vi "main.vi"() -> ()   [LabVIEW 2024, in "CLZ_to_ComicVine.lvlib"]
uses:
  CLZ_to_ComicVine.lvlib
  typedefs/CLZ_series.ctl
  comic_manager/manager_daemon/type_defs/VolumeData--cluster.ctl
  CV_Shared_Library/volume.type--enum.ctl
  <vilib>/addons/_JKI Toolkits/State Machine/_JKI_lib_State_Machine.llb/Select State(s)_err__jki_lib_state_machine.vi
  <vilib>/addons/_JKI Toolkits/State Machine/_JKI_lib_State_Machine.llb/Periodic Trigger__ogtk__JKI-SM__jki_lib_state_machine.vi
  CV_Shared_Library/CV_Shared_Library.lvlib
  comic_manager/manager_daemon/manager_daemon.lvclass
panel:
  in  "CV Volumes":i32(listbox)
  in  "CLZ Volumes":i32(listbox)
  in  "Load Files":bool
  in  "Exit":bool
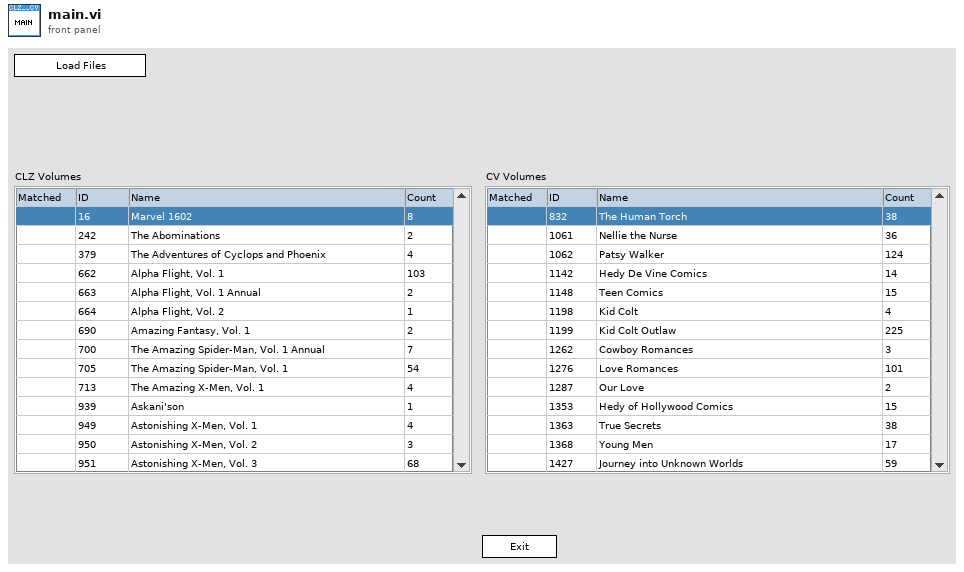
[diagram p1: front panel]
types:
  T1 = enum32{"Invalid", "Standard", "Closed", "Hidden", "Minimized", "Maximized"}
  T2 = enum32{"invalid app kind", "Development System", "Run Time System", "Student Edition", "Embedded LabVIEW", "Evaluation", "Custom"}
  T3 = typedef "CLZ_to_ComicVine.lvlib/CLZ_series.ctl" = cluster{"name":string, "id":i32, "earliest date":timestamp, "latest date":timestamp, "issue numbers":set{i32}}
  T4 = typedef "manager_daemon.lvclass/VolumeData--cluster.ctl" = cluster{"name":string, "sortable_name":string, "aliases":string[], "description":string, "site_detail_url":string, "count_of_issues":i32, "start_year":i32, "publisher_id":i32, "issue_ids":i32[], "date_last_updated":timestamp, "volume":i32, "cv_id":string, "volume type":T5, "source_path":path}
  T5 = typedef "CV_Shared_Library.lvlib/volume.type--enum.ctl" = enum16{"Ongoing", "Limited Series", "Annual", "One Shot", "Reprint/Document", "Star Comics", "Epic Comics"}
  T6 = cluster{"Core":cluster{"Current VI Reference":refnum<vi>, "Close Panel on Exit?":bool}, "CLZ report path":path, "clz series map":map{i32, T3}, "CV binary path":path, "cv volume map":map{i32, T4}, "matched volumes set":set{cluster{"CLZ ID":i32, "CV ID":i32}}}
  T7 = cluster{"Current VI Reference":refnum<vi>, "Close Panel on Exit?":bool}
  T8 = typedef "CLZ_to_ComicVine.lvlib/CLZ_comic.ctl" = cluster{"Series":string, "Core SeriesID":i32, "Core ComicID":i32, "Issue":string, "Issue Nr":i32, "Release Date":timestamp, "Barcode":string, "Cover Price":dbl, "CovrPrice Value":dbl, "Purchase Price":dbl, "Characters":string[]}
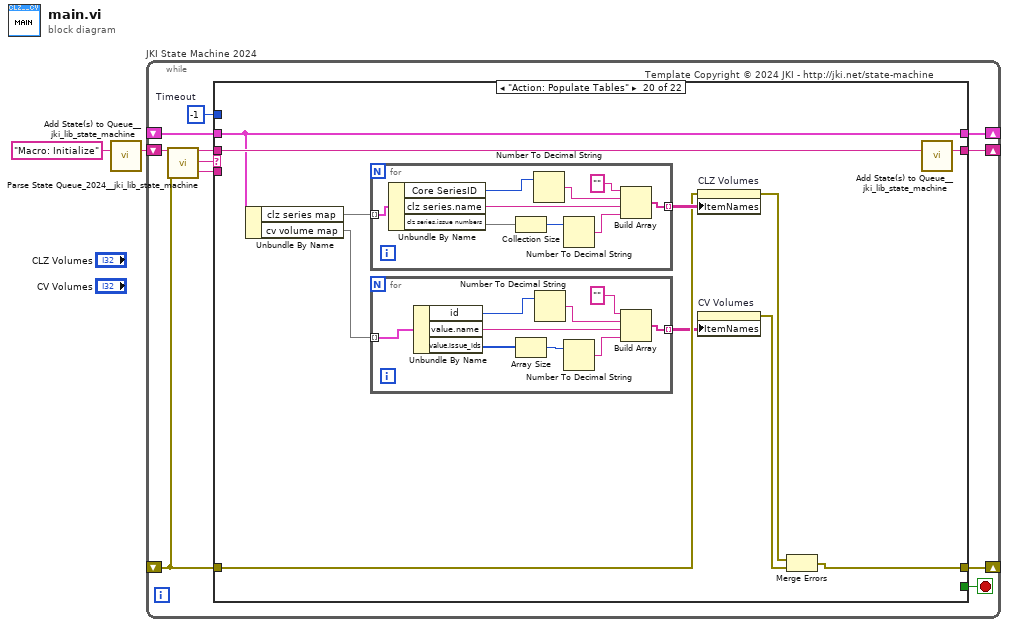
[diagram p0: block diagram]
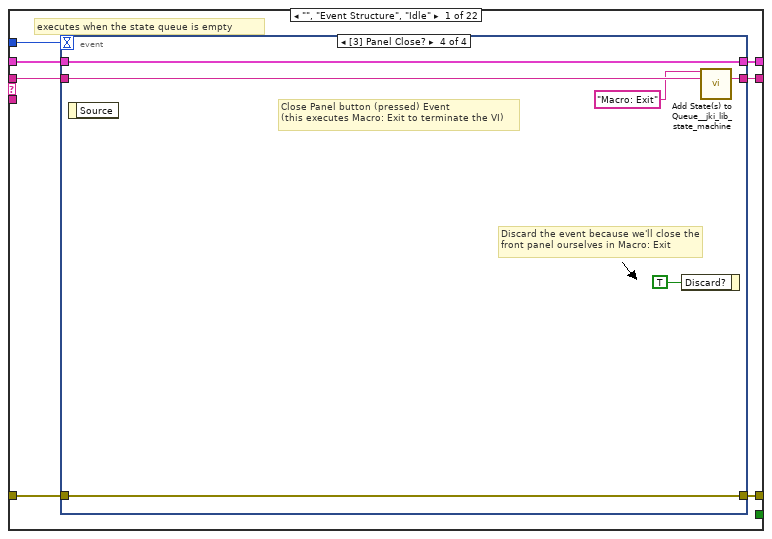
[diagram p2: hidden frame]
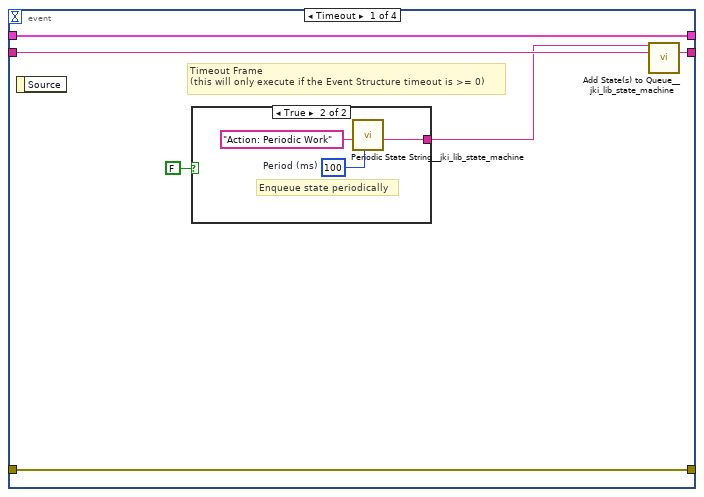
[diagram p3: hidden frame]
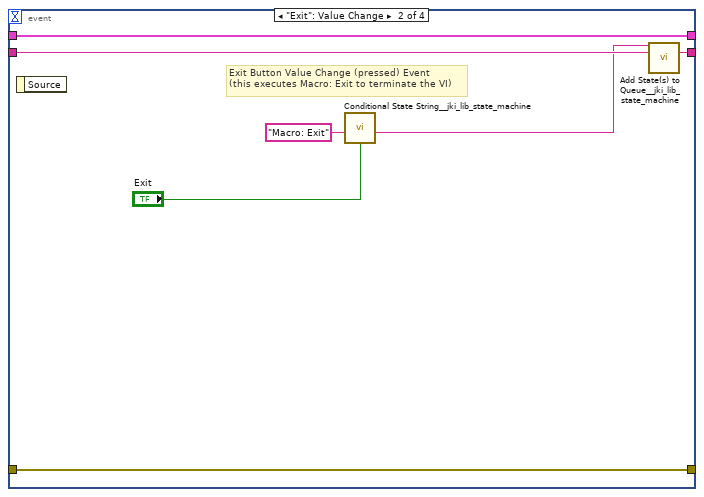
[diagram p5: hidden frame]
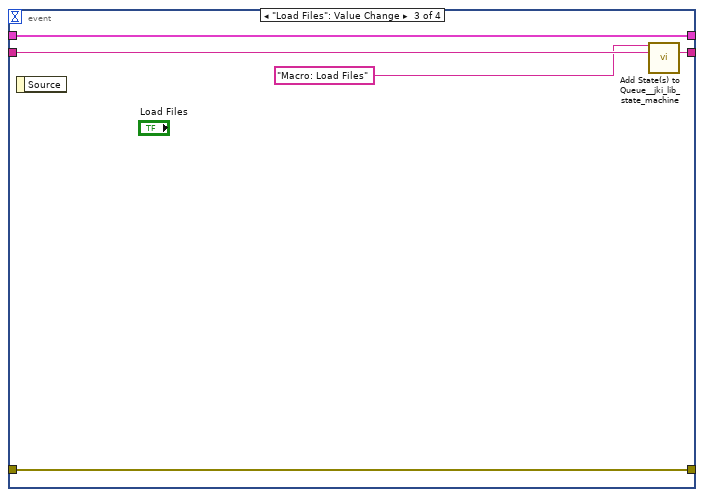
[diagram p6: hidden frame]
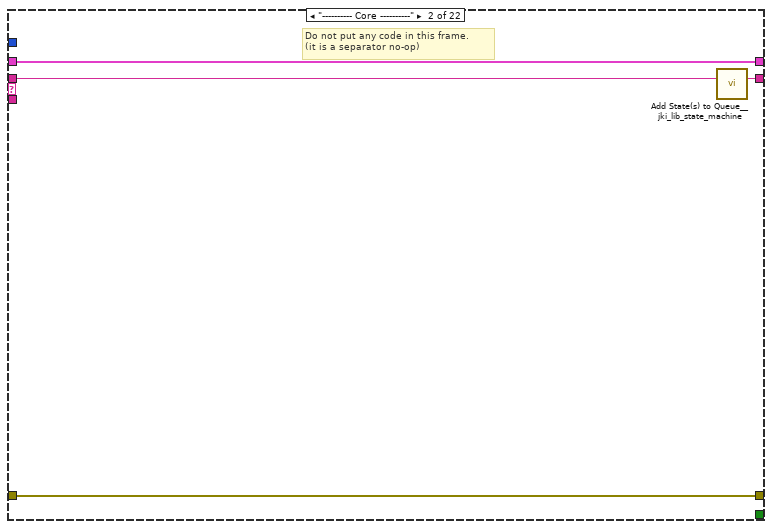
[diagram p7: hidden frame]
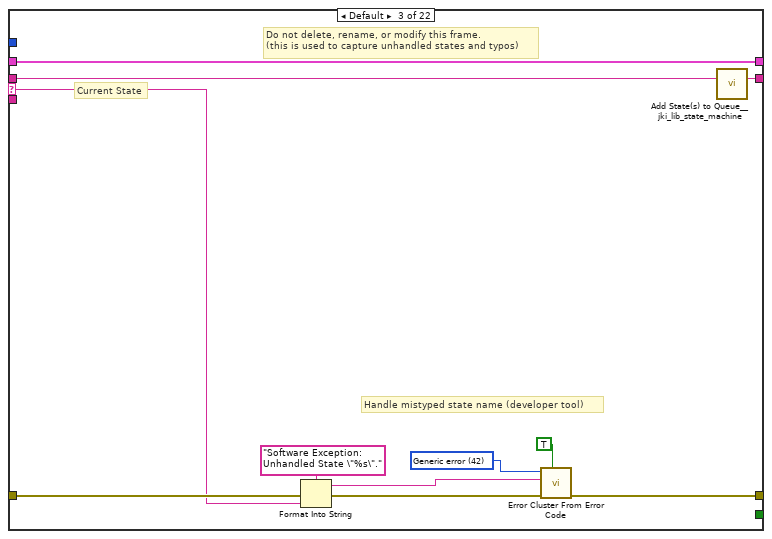
[diagram p8: hidden frame]
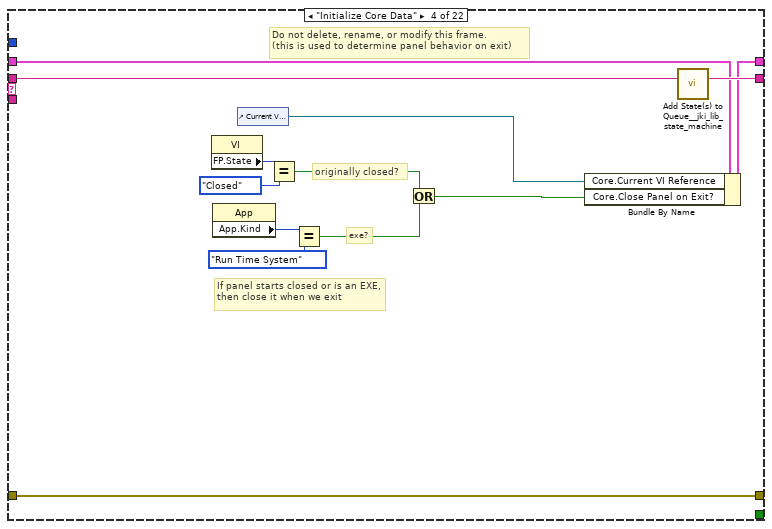
[diagram p9: hidden frame]
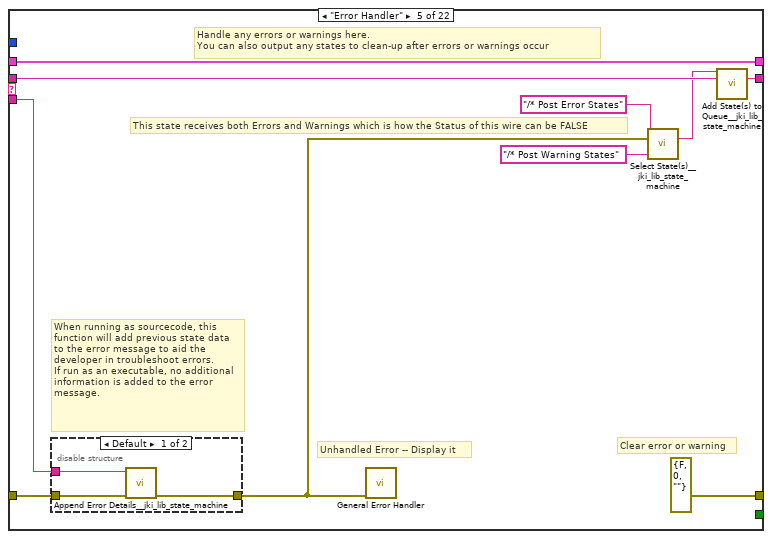
[diagram p10: hidden frame]
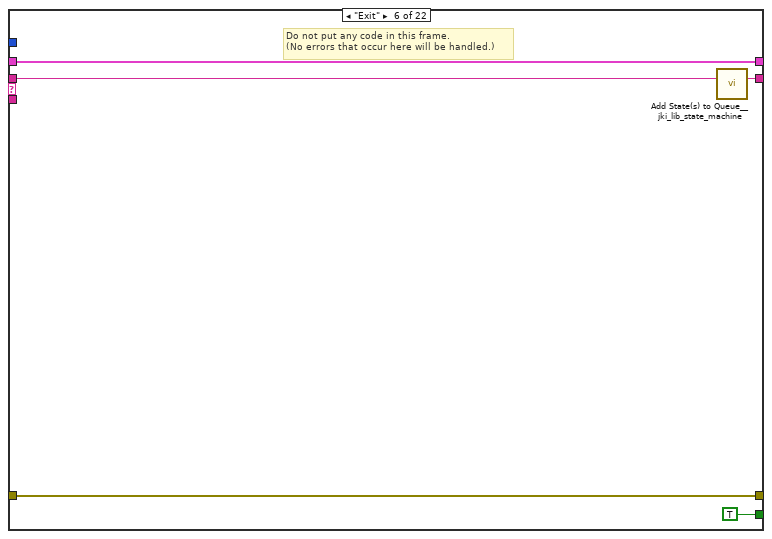
[diagram p12: hidden frame]
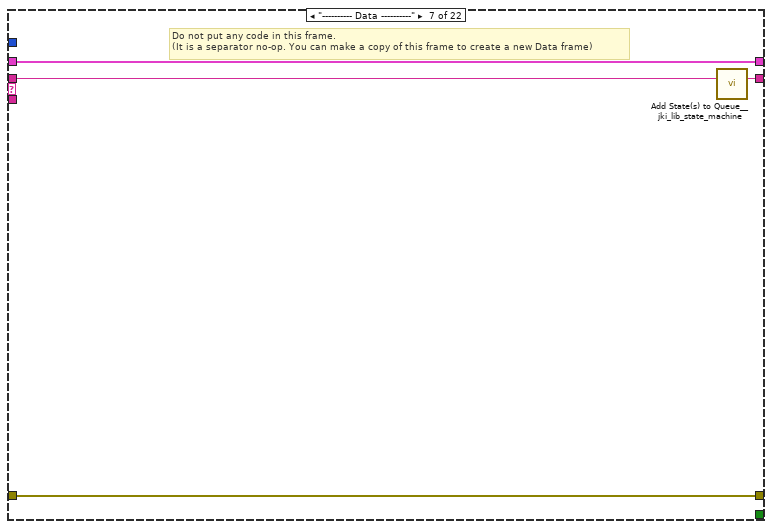
[diagram p13: hidden frame]
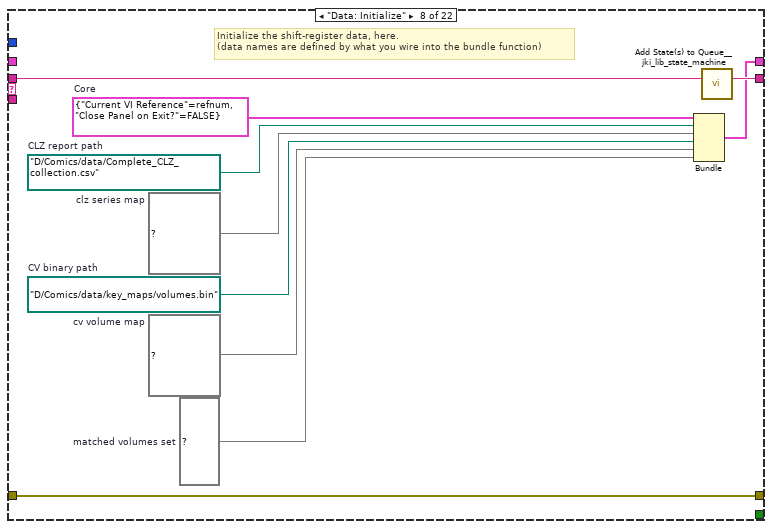
[diagram p14: hidden frame]
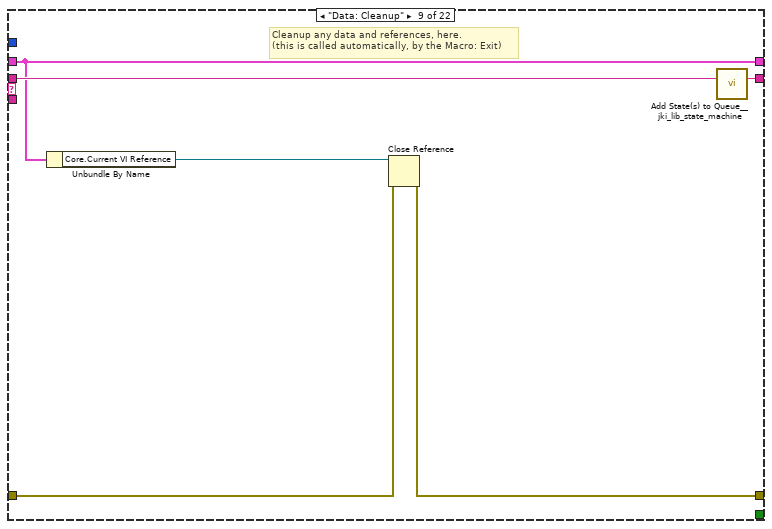
[diagram p15: hidden frame]
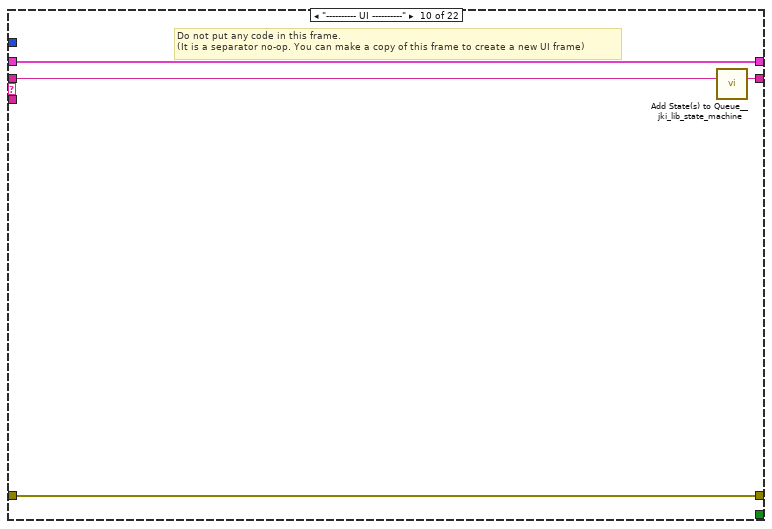
[diagram p16: hidden frame]
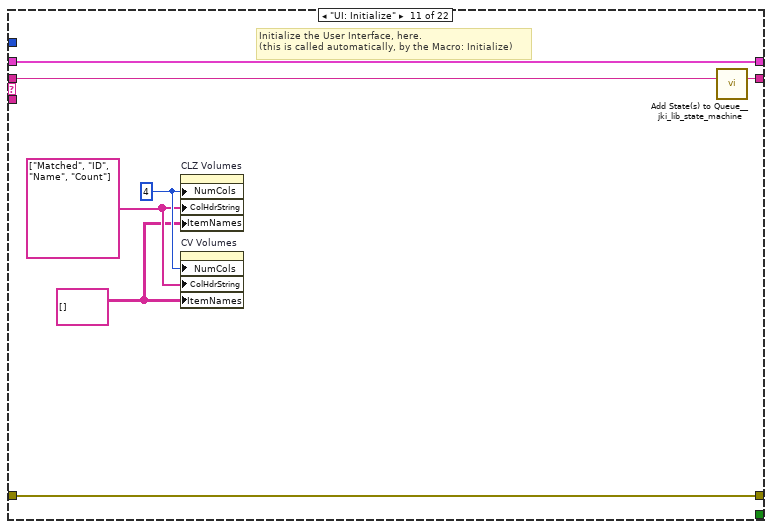
[diagram p17: hidden frame]
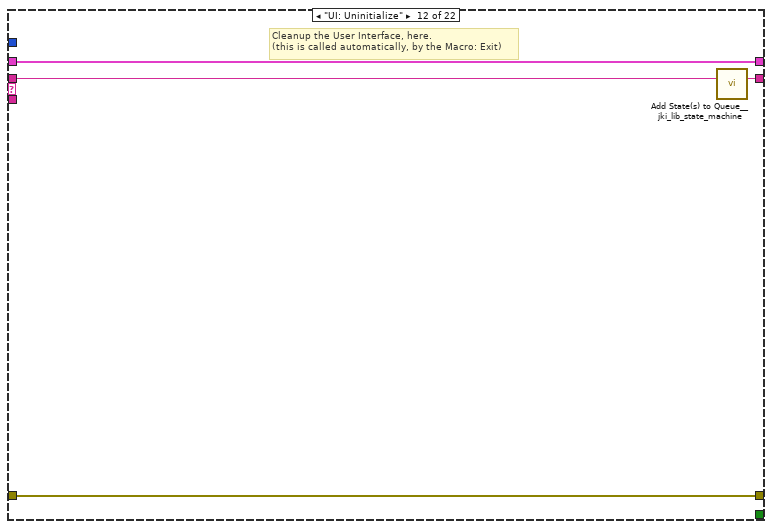
[diagram p18: hidden frame]
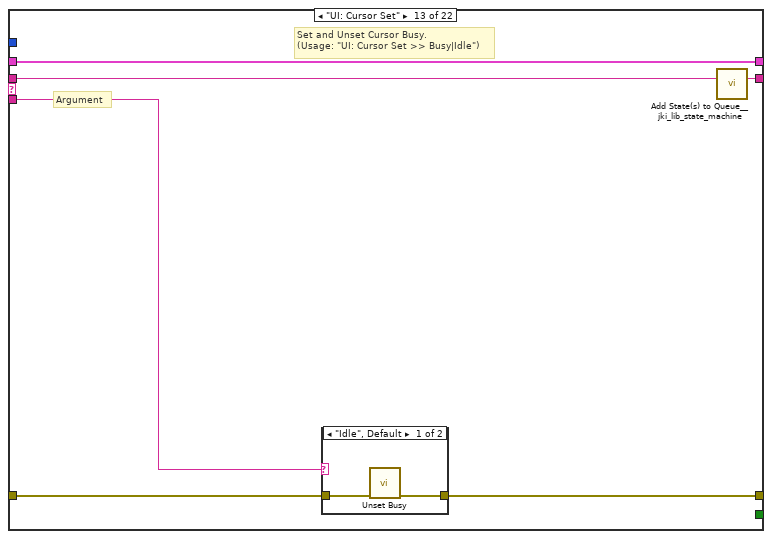
[diagram p19: hidden frame]
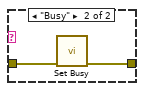
[diagram p20: hidden frame]
diagram:
  n1 = call <vilib>:"Add State(s) to Queue__jki_lib_state_machine.vi"("State(s) in (\"\")"="Macro: Initialize") -> ("States Out"=w2:string)  [unwired: 14 in]
  n2 = while "JKI State Machine 2024" {
    shift-right: [w6] -> _
    shift-left: _ -> [w5]
    shift-right: [w9] -> _
    shift-left: _ -> [w3]
    shift-right: [w8] -> _
    shift-left: w2 -> [w10]
    stop <- w7 stop-if-true
    w4 = -1  # Timeout
    # "Template Copyright © 2024 JKI - http://jki.net/state-machine"
    n3 = call <vilib>:"Parse State Queue_2024__jki_lib_state_machine.vi"("State Queue"=w10, "Error In (no error)"=w3) -> ("Remaining States"=w12:string, "Current State"=w13:string, "Arguments"=w11:string)  [unwired: 11 in]
    n4 = case shown="\"Action: Populate Tables\"" w13 {
      selector: w13 -> [_ _ w52 _ _ _ _ _ _ _ _ _ _ _ _ _ _ _ _ _ _ _]
      tunnel: w12 -> [w20 w51 w56 w75 w85 w94 w98 w108 w114 w118 w125 w129 w135 w146 w215 w220 w225 w234 w238 w249 w276 w282]
      tunnel: w11 -> [_ _ _ _ w80 _ _ _ _ _ _ _ w130 w140 _ _ _ _ _ _ _ _]
      tunnel: w5 -> [w18 w48 w54 w68 w82 w92 w95 _ w109 w115 w123 w127 w133 w142 w212 w217 w222 w232 w235 w247 w271 w280]
      tunnel: [w17 w49 w58 w72 errorcluster {"status"=FALSE, "code"=0, "source"=""} ("error out") w91 w96 w105 w110 w116 w122 w126 w131 w143 w213 w218 w223 w229 w236 w239 w273 w279] -> w9
      tunnel: w3 -> [w14 w49 w57 w72 w81 w91 w96 w105 w111 w116 w122 w126 w132 w144 w213 w218 w223 w229 w236 w244 w272 w278]
      tunnel: [w19 w50 w55 w74 w84 w93 w97 w107 w113 w117 w124 w128 w134 w145 w214 w219 w224 w233 w237 w248 w275 w281] -> w8
      tunnel: [_ _ _ _ _ TRUE _ _ _ _ _ _ _ _ _ _ _ _ _ _ _ _] -> w7
      tunnel: [w16 w48 w54 w73 w82 w92 w95 w106 w109 w115 w123 w127 w133 w142 w212 w217 w222 w232 w235 w247 w270 w277] -> w6
      tunnel: w4 -> [w15 _ _ _ _ _ _ _ _ _ _ _ _ _ _ _ _ _ _ _ _ _]
      frame "", "Event Structure", "Idle" {
        # "executes when the state queue is empty"
        n5 = event shown="[3] Panel Close?" {
          selector: _ -> [_ _ _ _]
          dyn-events: _ -> [_ _ _ _]
          timeout: w15 -> [_ _ _ _]
          tunnel: w20 -> [w26 w36 w41 w47]
          tunnel: [w25 w35 w40 w46] -> w19
          tunnel: w18 -> [w23 w33 w38 w44]
          tunnel: [w24 w34 w39 w45] -> w17
          tunnel: w14 -> [w24 w34 w39 w45]
          tunnel: [w23 w33 w38 w44] -> w16
          event Timeout {
            # "Timeout Frame\n(this will only execute if the Event Structure timeout is >= 0)"
            n6 = event-data() -> ()  [unwired: 1 in, 1 out]
            n7 = case shown="True" FALSE {
              tunnel: [_ w29] -> w22
              frame False {
              }
              frame True {
                w27 = u32 100  # Period (ms)
                # "Enqueue state periodically"
                n8 = call <vilib>:"Periodic State String__jki_lib_state_machine.vi"("Period (ms)"=w27, "State"="Action: Periodic Work") -> ("State Out"=w29:string)  [unwired: 9 in]
              }
            }
            n9 = call <vilib>:"Add State(s) to Queue__jki_lib_state_machine.vi"("State(s) in Front (\"\")"=w22, "State(s) in (\"\")"=w26) -> ("States Out"=w25:string)  [unwired: 13 in]
          }
          event "Exit": Value Change {
            # "Exit Button Value Change (pressed) Event\n(this executes Macro: Exit to terminate the VI)"
            n10 = event-data() -> ()  [unwired: 1 in, 1 out]
            n11 = call <vilib>:"Conditional State String__jki_lib_state_machine.vi"("Do State(s)?"="Exit", "State"="Macro: Exit") -> ("State Out"=w30:string)  [unwired: 7 in]
            n12 = call <vilib>:"Add State(s) to Queue__jki_lib_state_machine.vi"("State(s) in Front (\"\")"=w30, "State(s) in (\"\")"=w36) -> ("States Out"=w35:string)  [unwired: 13 in]
          }
          event "Load Files": Value Change {
            n13 = event-data() -> ()  [unwired: 1 in, 1 out]
            n14 = call <vilib>:"Add State(s) to Queue__jki_lib_state_machine.vi"("State(s) in Front (\"\")"="Macro: Load Files", "State(s) in (\"\")"=w41) -> ("States Out"=w40:string)  [unwired: 13 in]
          }
          event Panel Close? {
            # "Discard the event because we'll close the front panel ourselves in Macro: Exit"
            # "Close Panel button (pressed) Event\n(this executes Macro: Exit to terminate the VI)"
            n15 = event-data() -> ()  [unwired: 1 in, 1 out]
            n16 = event-data("Discard?"=TRUE) -> ()  [unwired: 1 in, 1 out]
            n17 = call <vilib>:"Add State(s) to Queue__jki_lib_state_machine.vi"("State(s) in Front (\"\")"="Macro: Exit", "State(s) in (\"\")"=w47) -> ("States Out"=w46:string)  [unwired: 13 in]
          }
        }
      }
      frame "---------- Core ----------" {
        # "Do not put any code in this frame.\n(it is a separator no-op)"
        n18 = call <vilib>:"Add State(s) to Queue__jki_lib_state_machine.vi"("State(s) in (\"\")"=w51) -> ("States Out"=w50:string)  [unwired: 14 in]
      }
      frame Default {
        w61 = 42 items=["No error", "Argument error", "Memory is full", "Out of zone", "End of file", "File already open", "Generic file I/O error", "File not found", "File permission error", "Disk is full", "Duplicate path", "Too many files open", "System feature not enabled", "Resource file not found", "Cannot add resource", "Resource not found", "Image not found", "Image memory error", "Pen does not exist", "Config type invalid", "Config token not found", "Config parse error", "Config memory error", "Bad external code format", "Bad external code offset", "External code not present", "Null window", "Destroy window error", "Null menu", "Print aborted", "Bad print record", "Print driver error", "Windows error during printing", "Memory error during printing", "Print dialog error", "Generic print error", "Invalid device refnum", "Device not found", "Device parameter error", "Device unit error", "Cannot open device", "Device call aborted", "Generic error", "Cancelled by user", "Object ID too low", "Object ID too high", "Object not in heap", "Unknown heap", "Unknown object (invalid DefProc)", "Unknown object (DefProc not in table)", "Message out of range", "Invalid (null) method", "Unknown message", "Manager call not supported", "Bad address", "Network operation in progress", "Network operation timed out", "Connection is busy", "Network attribute not supported", "Network error", "Address in use", "System out of memory", "Connection aborted", "Connection refused", "Not connected", "Already connected", "Connection closed", "Initialization error (interapplication manager)", "Bad occurrence", "Wait on unbound occurrence handler", "Occurrence queue overflow", "Datalog type conflict", "Unused", "Unrecognized type (interapplication manager)", "Memory corrupt", "Failed to make temporary DLL", "Old CIN version", "Drag socket not found", "Failed to load drop-object", "Failed to register OLE object", "Failed to release OLE object", "Format specifier type mismatch", "Unknown format specifier", "Too few format specifiers", "Too many format specifiers", "Scan failed", "Newer CIN version", "Error converting to variant", "Runtime menu error", "Password tampered", "Variant attribute not found", "Incompatible variant data type", "Event data is not available", "Event Store is not present", "Occurrence is not found", "Event Queue is not created", "Event info is not available", "Refnum passed is NULL", "Error retrieving Class GUID", "Error retrieving CoClass GUID", "Error retrieving TypeLib GUID.", "Bad built application magic bytes.", "Specific driver is different from the specific driver associated with the Logical Name.", "There is no session opened to the class driver.", "Max Error", "MAX - Error with config objects", "MAX - Error loading configuration", "MAX - Group not supported"]
        # "Current State"
        # "Do not delete, rename, or modify this frame.\n(this is used to capture unhandled states and typos)"
        # "Handle mistyped state name (developer tool)"
        n19 = Format Into String(format string="Software Exception: Unhandled State \"%s\"." ("message"), error in=w57, w52) -> (resulting string=w60:string, error out=w59:errorcluster)  [unwired: 1 in]
        n20 = call <vilib>:"Error Cluster From Error Code.vi"("show call chain? (False)"=TRUE, "error in (no error)"=w59, "error message (\"\")"=w60, "error code (0)"=w61) -> ("error out"=w58:errorcluster)  [unwired: 5 in]
        n21 = call <vilib>:"Add State(s) to Queue__jki_lib_state_machine.vi"("State(s) in (\"\")"=w56) -> ("States Out"=w55:string)  [unwired: 14 in]
      }
      frame "Initialize Core Data" {
        # "Do not delete, rename, or modify this frame.\n(this is used to determine panel behavior on exit)"
        # "originally closed?"
        # "exe?"
        # "If panel starts closed or is an EXE, then close it when we exit"
        n22 = property class="VI"() -> ("FP.State"=w65:T1)  [unwired: 2 in, 2 out]
        n23 = property class="App"() -> ("App.Kind"=w71:T2)  [unwired: 2 in, 2 out]
        n24 = control-ref of="Current VI Reference"() -> (w66:refnum<vi>)
        n25 = Equal?(x=w65, y=T1."Closed" ("Front Panel Window:State")) -> (x = y?=w63:bool)
        n26 = Equal?(x=w71, y=T2."Run Time System" ("Application:Kind")) -> (x = y?=w69:bool)
        n27 = Or(x=w63, y=w69) -> (x .or. y?=w67:bool)
        n28 = Bundle By Name(cluster=w68, "Core.Current VI Reference"=w66, "Core.Close Panel on Exit?"=w67) -> (w73:T6)
        n29 = call <vilib>:"Add State(s) to Queue__jki_lib_state_machine.vi"("State(s) in (\"\")"=w75) -> ("States Out"=w74:string)  [unwired: 14 in]
      }
      frame "Error Handler" {
        # "When running as sourcecode, this function will add previous state data to the error message to aid the developer in troubleshoot errors.\nIf run as an executable, no additional information is added to the error message."
        # "This state receives both Errors and Warnings which is how the Status of this wire can be FALSE"
        # "Unhandled Error -- Display it"
        # "Handle any errors or warnings here.\nYou can also output any states to clean-up after errors or warnings occur"
        # "Clear error or warning"
        n30 = disable-structure shown="Default" {
          disable-tunnel: w81 -> [w88 w89]
          disable-tunnel: w80 -> [w87 _]
          disable-tunnel: [w86 w89] -> w79
          frame condition #0 (active) {
            n31 = call <vilib>:"Append Error Details__jki_lib_state_machine.vi"("error in (no error)"=w88, "Previous State and Argument(s)"=w87) -> ("error out"=w86:errorcluster)  [unwired: 9 in]
          }
          frame condition #1 {
          }
        }
        n32 = call <vilib>:"General Error Handler.vi"("error in (no error)"=w79) -> ()  [unwired: 10 in, 5 out]
        n33 = call-poly <vilib>:"Select State(s)__jki_lib_state_machine.vi"("State(s) if True (\"\")"="/* Post Error States", "Select"=w79, "State(s) if False (\"\")"="/* Post Warning States") -> ("States Out"=w77:string)  [unwired: 12 in]
        n34 = call <vilib>:"Add State(s) to Queue__jki_lib_state_machine.vi"("State(s) in Front (\"\")"=w77, "State(s) in (\"\")"=w85) -> ("States Out"=w84:string)  [unwired: 13 in]
      }
      frame "Exit" {
        # "Do not put any code in this frame.\n(No errors that occur here will be handled.)"
        n35 = call <vilib>:"Add State(s) to Queue__jki_lib_state_machine.vi"("State(s) in (\"\")"=w94) -> ("States Out"=w93:string)  [unwired: 14 in]
      }
      frame "---------- Data ----------" {
        # "Do not put any code in this frame.\n(It is a separator no-op. You can make a copy of this frame to create a new Data frame)"
        n36 = call <vilib>:"Add State(s) to Queue__jki_lib_state_machine.vi"("State(s) in (\"\")"=w98) -> ("States Out"=w97:string)  [unwired: 14 in]
      }
      frame "Data: Initialize" {
        w99 = set{cluster{"CLZ ID":i32, "CV ID":i32}} {}  # matched volumes set
        w100 = map{i32, T4} {}  # cv volume map
        w101 = path "D:/Comics/data/key_maps/volumes.bin"  # CV binary path
        w102 = map{i32, T3} {}  # clz series map
        w103 = path "D:/Comics/data/Complete_CLZ_collection.csv"  # CLZ report path
        w104 = T7 {"Current VI Reference"=refnum, "Close Panel on Exit?"=FALSE}  # Core
        # "Initialize the shift-register data, here.\n(data names are defined by what you wire into the bundle function)"
        n37 = Bundle("Core"=w104, "CLZ report path"=w103, "clz series map"=w102, "CV binary path"=w101, "cv volume map"=w100, "matched volumes set"=w99) -> (w106:T6)  [unwired: 1 in]
        n38 = call <vilib>:"Add State(s) to Queue__jki_lib_state_machine.vi"("State(s) in (\"\")"=w108) -> ("States Out"=w107:string)  [unwired: 14 in]
      }
      frame "Data: Cleanup" {
        # "Cleanup any data and references, here.\n(this is called automatically, by the Macro: Exit)"
        n39 = Unbundle By Name(w109) -> ("Core.Current VI Reference"=w112:refnum<vi>)
        n40 = Close Reference(reference=w112, error in (no error)=w111) -> (error out=w110:errorcluster)
        n41 = call <vilib>:"Add State(s) to Queue__jki_lib_state_machine.vi"("State(s) in (\"\")"=w114) -> ("States Out"=w113:string)  [unwired: 14 in]
      }
      frame "---------- UI ----------" {
        # "Do not put any code in this frame.\n(It is a separator no-op. You can make a copy of this frame to create a new UI frame)"
        n42 = call <vilib>:"Add State(s) to Queue__jki_lib_state_machine.vi"("State(s) in (\"\")"=w118) -> ("States Out"=w117:string)  [unwired: 14 in]
      }
      frame "UI: Initialize" {
        w119 = string[][] []
        w120 = string[] ["Matched", "ID", "Name", "Count"] ("Row Header Strings[]")
        w121 = u32 4 ("Number of Columns")
        # "Initialize the User Interface, here.\n(this is called automatically, by the Macro: Initialize)"
        n43 = property on="CLZ Volumes" class="MCListbox (strict)"("NumCols"=w121, "ColHdrString"=w120, "ItemNames"=w119) -> ()  [unwired: 2 in, 2 out]
        n44 = property on="CV Volumes" class="MCListbox (strict)"("NumCols"=w121, "ColHdrString"=w120, "ItemNames"=w119) -> ()  [unwired: 2 in, 2 out]
        n45 = call <vilib>:"Add State(s) to Queue__jki_lib_state_machine.vi"("State(s) in (\"\")"=w125) -> ("States Out"=w124:string)  [unwired: 14 in]
      }
      frame "UI: Uninitialize" {
        # "Cleanup the User Interface, here.\n(this is called automatically, by the Macro: Exit)"
        n46 = call <vilib>:"Add State(s) to Queue__jki_lib_state_machine.vi"("State(s) in (\"\")"=w129) -> ("States Out"=w128:string)  [unwired: 14 in]
      }
      frame "UI: Cursor Set" {
        # "Argument"
        # "Set and Unset Cursor Busy.\n(Usage: \"UI: Cursor Set >> Busy|Idle\")"
        n47 = case shown="\"Idle\", Default" w130 {
          tunnel: w132 -> [w137 w139]
          tunnel: [w136 w138] -> w131
          frame "Idle", Default {
            n48 = call <vilib>:"Unset Busy.vi"("error in (no error)"=w137) -> ("error out"=w136:errorcluster)  [unwired: 10 in]
          }
          frame "Busy" {
            n49 = call <vilib>:"Set Busy.vi"("error in (no error)"=w139) -> ("error out"=w138:errorcluster)  [unwired: 9 in, 1 out]
          }
        }
        n50 = call <vilib>:"Add State(s) to Queue__jki_lib_state_machine.vi"("State(s) in (\"\")"=w135) -> ("States Out"=w134:string)  [unwired: 14 in]
      }
      frame "UI: Front Panel State" {
        # "Argument"
        # "Set Front Panel Open or Closed\n(Usage: \"UI: Front Panel State >> Open|Close\")"
        n51 = Unbundle By Name(w142) -> ("Core.Current VI Reference"=w141:refnum<vi>)
        n52 = case shown="\"Minimize\", \"Minimized\"" w140 {
          tunnel: w144 -> [w152 w167 w178 w191 w204]
          tunnel: [w154 w168 w180 w193 w206] -> w143
          tunnel: w141 -> [w153 w165 w179 w192 w205]
          frame "Open", "Standard", Default {
            w147 = T1."Standard" ("State")
            n53 = property class="VI"(reference=w153, error in=w152) -> (reference out=w150:refnum<vi>, error out=w151:errorcluster, "FP.State"=w149:T1)
            n54 = Not Equal?(x=w149, y=w147) -> (x != y?=w148:bool)
            n55 = case shown="True" w148 {
              tunnel: [w158 w160] -> w154
              tunnel: w151 -> [w157 w160]
              tunnel: w150 -> [w156 _]
              tunnel: w147 -> [w155 _]
              frame True {
                n56 = invoke class="VI" method="FP.Open"(reference=w156, error in=w157, "Activate"=TRUE, "State"=w155) -> (error out=w158:errorcluster)  [unwired: 1 in, 4 out]
              }
              frame False {
              }
            }
          }
          frame "Close", "Closed" {
            n57 = property class="VI"(reference=w165, error in=w167) -> (reference out=w164:refnum<vi>, error out=w166:errorcluster, "FP.State"=w162:T1)
            n58 = Not Equal?(x=w162, y=T1."Closed" ("Front Panel Window:State")) -> (x != y?=w161:bool)
            n59 = case shown="True" w161 {
              tunnel: [w169 w172] -> w168
              tunnel: w166 -> [w169 w171]
              tunnel: w164 -> [_ w170]
              frame False {
              }
              frame True {
                n60 = invoke class="VI" method="FP.Close"(reference=w170, error in=w171) -> (error out=w172:errorcluster)  [unwired: 1 in, 2 out]
              }
            }
          }
          frame "Hidden", "Hide" {
            w173 = T1."Hidden" ("State")
            n61 = property class="VI"(reference=w179, error in=w178) -> (reference out=w176:refnum<vi>, error out=w177:errorcluster, "FP.State"=w175:T1)
            n62 = Not Equal?(x=w175, y=w173) -> (x != y?=w174:bool)
            n63 = case shown="True" w174 {
              tunnel: [w184 w185] -> w180
              tunnel: w177 -> [w183 w185]
              tunnel: w176 -> [w182 _]
              tunnel: w173 -> [w181 _]
              frame True {
                n64 = invoke class="VI" method="FP.Open"(reference=w182, error in=w183, "State"=w181) -> (error out=w184:errorcluster)  [unwired: 2 in, 4 out]
              }
              frame False {
              }
            }
          }
          frame "Minimize", "Minimized" {
            w186 = T1."Minimized" ("State")
            n65 = property class="VI"(reference=w192, error in=w191) -> (reference out=w189:refnum<vi>, error out=w190:errorcluster, "FP.State"=w188:T1)
            n66 = Not Equal?(x=w188, y=w186) -> (x != y?=w187:bool)
            n67 = case shown="True" w187 {
              tunnel: [w197 w198] -> w193
              tunnel: w190 -> [w196 w198]
              tunnel: w189 -> [w195 _]
              tunnel: w186 -> [w194 _]
              frame True {
                n68 = invoke class="VI" method="FP.Open"(reference=w195, error in=w196, "State"=w194) -> (error out=w197:errorcluster)  [unwired: 2 in, 4 out]
              }
              frame False {
              }
            }
          }
          frame "Maximize", "Maximized" {
            w199 = T1."Maximized" ("State")
            n69 = property class="VI"(reference=w205, error in=w204) -> (reference out=w202:refnum<vi>, error out=w203:errorcluster, "FP.State"=w201:T1)
            n70 = Not Equal?(x=w201, y=w199) -> (x != y?=w200:bool)
            n71 = case shown="True" w200 {
              tunnel: [w210 w211] -> w206
              tunnel: w203 -> [w209 w211]
              tunnel: w202 -> [w208 _]
              tunnel: w199 -> [w207 _]
              frame True {
                n72 = invoke class="VI" method="FP.Open"(reference=w208, error in=w209, "State"=w207) -> (error out=w210:errorcluster)  [unwired: 2 in, 4 out]
              }
              frame False {
              }
            }
          }
        }
        n73 = call <vilib>:"Add State(s) to Queue__jki_lib_state_machine.vi"("State(s) in (\"\")"=w146) -> ("States Out"=w145:string)  [unwired: 14 in]
      }
      frame "---------- Macro ----------" {
        # "Do not put any code in this frame.\n(It is a separator no-op. You can make a copy of this frame to create a new Macro frame)"
        n74 = call <vilib>:"Add State(s) to Queue__jki_lib_state_machine.vi"("State(s) in (\"\")"=w215) -> ("States Out"=w214:string)  [unwired: 14 in]
      }
      frame "Macro: Initialize" {
        w216 = "Data: Initialize\nInitialize Core Data\nUI: Initialize\nUI: Front Panel State >> Open"  # Data: Initialize Initialize Core Data UI: Initialize UI: Front Panel State >> Open
        # "Initialization Macro\n(This is called once, when the VI starts)"
        n75 = call <vilib>:"Add State(s) to Queue__jki_lib_state_machine.vi"("State(s) in Front (\"\")"=w216, "State(s) in (\"\")"=w220) -> ("States Out"=w219:string)  [unwired: 13 in]
      }
      frame "Macro: Load Files" {
        n76 = call <vilib>:"Add State(s) to Queue__jki_lib_state_machine.vi"("State(s) in Front (\"\")"="UI: Cursor Set >> Busy\nAction: Load CLZ Report\nAction: Load CV Binary\nAction: Populate Tables\nUI: Cursor Set >> Idle", "State(s) in (\"\")"=w225) -> ("States Out"=w224:string)  [unwired: 13 in]
      }
      frame "Macro: Exit" {
        # "Exit Macro\n(This is called once, when the VI exits)"
        n77 = Unbundle By Name(w232) -> ("Core.Close Panel on Exit?"=w227:bool)
        n78 = call <vilib>:"Conditional State String__jki_lib_state_machine.vi"("Do State(s)?"=w227, "State"="UI: Front Panel State >> Close") -> ("State Out"=w226:string)  [unwired: 7 in]
        n79 = call <vilib>:"Add State(s) to Queue__jki_lib_state_machine.vi"("State(s) in (\"\")"=w226, "State(s) at Back (\"\")"="UI: Uninitialize\nData: Cleanup\nExit") -> ("States Out"=w230:string)  [unwired: 13 in]
        n80 = call <vilib>:"Add State(s) to Queue__jki_lib_state_machine.vi"("State(s) in Front (\"\")"=w230, "State(s) in (\"\")"=w234) -> ("States Out"=w233:string)  [unwired: 13 in]
      }
      frame "---------- Action ----------" {
        n81 = call <vilib>:"Add State(s) to Queue__jki_lib_state_machine.vi"("State(s) in (\"\")"=w238) -> ("States Out"=w237:string)  [unwired: 14 in]
      }
      frame "Action: Populate Tables" {
        n82 = Unbundle By Name(w247) -> ("clz series map"=w246:map{i32, T3}, "cv volume map"=w243:map{i32, T4})
        n83 = for {
          tunnel: w246 -> [w267] mode=indexing
          tunnel: [w262] -> w245 mode=indexing
          n84 = Unbundle By Name(w267) -> ("Core SeriesID"=w260:i32, "clz series.name"=w263:string, "clz series.issue numbers"=w266:set{i32})
          n85 = Collection Size(1:w266) -> (0:w265:i32)
          n86 = Number To Decimal String(number=w260) -> (decimal integer string=w259:string)  [unwired: 1 in]
          n87 = Number To Decimal String(number=w265) -> (decimal integer string=w264:string)  [unwired: 1 in]
          n88 = Build Array("" ("element"), w259, w263, w264) -> (w262:string[])
        }
        n89 = for {
          tunnel: w243 -> [w258] mode=indexing
          tunnel: [w253] -> w242 mode=indexing
          n90 = Unbundle By Name(w258) -> ("id"=w251:i32, "value.name"=w254:string, "value.issue_ids"=w257:i32[])
          n91 = Array Size(array=w257) -> (size(s)=w256:i32)
          n92 = Number To Decimal String(number=w251) -> (decimal integer string=w250:string)  [unwired: 1 in]
          n93 = Number To Decimal String(number=w256) -> (decimal integer string=w255:string)  [unwired: 1 in]
          n94 = Build Array("" ("element"), w250, w254, w255) -> (w253:string[])
        }
        n95 = property on="CLZ Volumes" class="MCListbox (strict)"(error in=w244, "ItemNames"=w245) -> (error out=w241:errorcluster)  [unwired: 1 in, 1 out]
        n96 = property on="CV Volumes" class="MCListbox (strict)"("ItemNames"=w242) -> (error out=w240:errorcluster)  [unwired: 2 in, 1 out]
        n97 = Merge Errors(w241, w240) -> (w239:errorcluster)
        n98 = call <vilib>:"Add State(s) to Queue__jki_lib_state_machine.vi"("State(s) in (\"\")"=w249) -> ("States Out"=w248:string)  [unwired: 14 in]
      }
      frame "Action: Load CLZ Report" {
        n99 = Unbundle By Name(w271) -> ("CLZ report path"=w274:path)
        n100 = call "load_full_report.vi"("error in (no error)"=w272, "report path"=w274) -> ("error out"=w273:errorcluster, "clz_comics"=w269:T8[])  [unwired: 8 in]
        n101 = call "parse_clz_series.vi"("clz comics"=w269) -> ("clz series map"=w268:map{i32, T3})  [unwired: 10 in]
        n102 = Bundle By Name(cluster=w271, "clz series map"=w268) -> (w270:T6)
        n103 = call <vilib>:"Add State(s) to Queue__jki_lib_state_machine.vi"("State(s) in (\"\")"=w276) -> ("States Out"=w275:string)  [unwired: 14 in]
      }
      frame "Action: Load CV Binary" {
        n104 = in-place {
          in-place-border: w278 -> [w287]
          in-place-border: [w284] -> w279
          n105 = in-place-cluster #1(w280) -> ("CV binary path"=w285:path, "cv volume map"=w286:map{i32, T4})
          n106 = Read from Binary File(5:w286, 8:w287, 11:w285) -> (0:w284:errorcluster, 2:w283:map{i32, T4})  [unwired: 3 in, 2 out]
          n107 = in-place-cluster #1("CV binary path"=w285, "cv volume map"=w283) -> (w277:T6)
          n108 = call "search_cv.vi"("data"=w283) -> ()  [unwired: 11 in]
        }
        n109 = call <vilib>:"Add State(s) to Queue__jki_lib_state_machine.vi"("State(s) in (\"\")"=w282) -> ("States Out"=w281:string)  [unwired: 14 in]
      }
    }
  }
